vi "CalculateFloatB.vi"(9 "sinHalfTheta":dbl, 10 "HalfTheta":dbl, 11 "t":dbl) -> (3 "FloatRatioB":dbl)   [LabVIEW 2015]
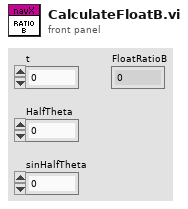
[diagram p1: front panel]
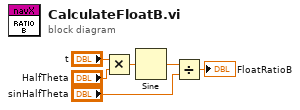
[diagram p0: block diagram]
diagram:
  n1 = Multiply(x="t", y="HalfTheta") -> (x*y=w2:dbl)
  n2 = Sine(x=w2) -> (sin(x)=w1:dbl)
  n3 = Divide(x=w1, y="sinHalfTheta") -> (x/y=→"FloatRatioB":dbl)
